vi "RSZVB Write Memory Trace Data Extended.vi"(6 "Trace Data":dbl[](array[numeric]) format="%^.3e", 7 "No of Points":i32, 8 "error in (no error)":errorcluster {"code" format="%.0x"}, 9 "Data Format (0: Unformatted)":i32(ring) items=["Unformatted", "Formatted", "Unformatted With Trace Mathematics"], 10 "Channel (Trace) (1)":i32=1, 11 "VISA session":refnum<visa-resource-name>) -> (0 "error out":errorcluster {"code" format="%.0x"}, 3 "dup VISA session":refnum<visa-resource-name>)   [LabVIEW 2011]
doc: "This VI writes a memory trace data to the instrument.\n\nRemote-control command(s):\nCALCulate<Chn>:DATA FDATa | SDATa | MDATa, <data>\nFORMat ASCII\nFORMat REAL,32\nSYSTem:COMMunicate:GPIB:SELF:RTERminator EOI"
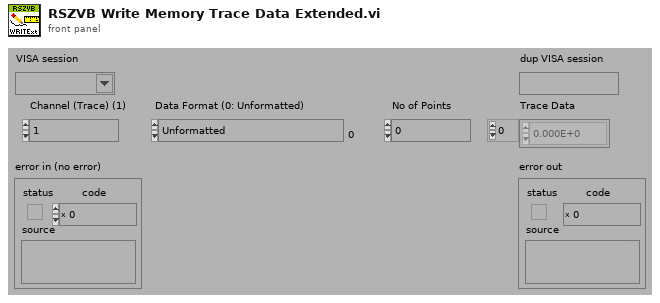
[diagram p1: front panel]
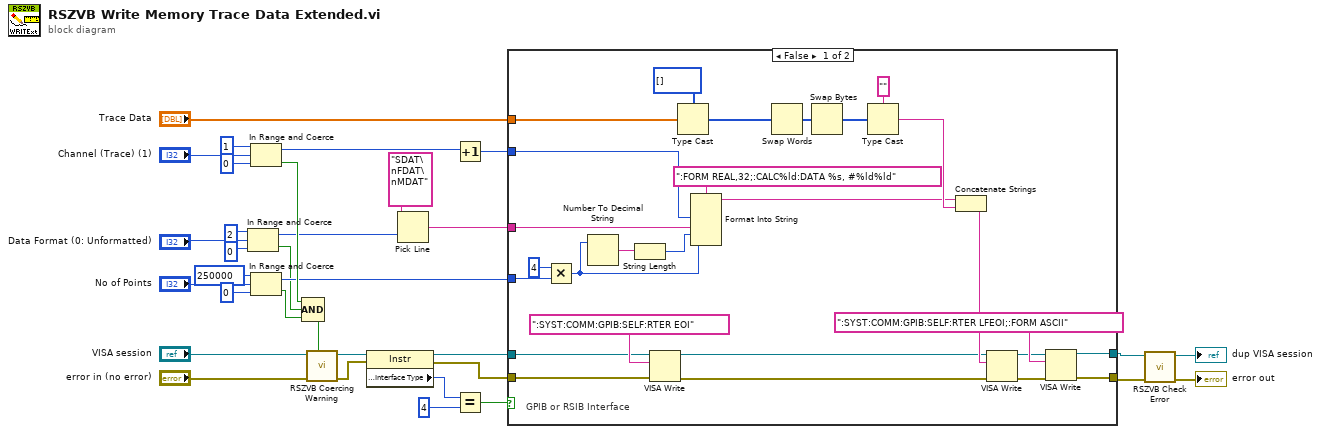
[diagram p0: block diagram]
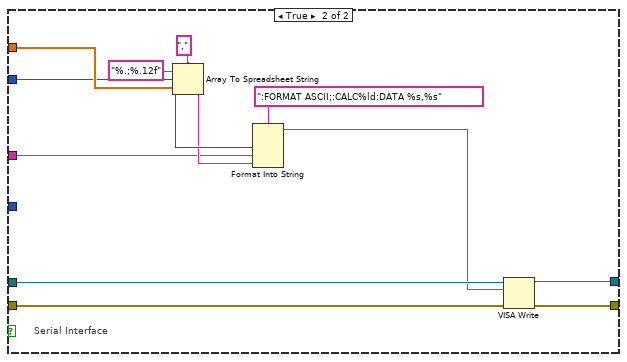
[diagram p2: hidden frame]
diagram:
  n1 = In Range and Coerce(upper limit=2, x="Data Format (0: Unformatted)", lower limit=0) -> (coerced(x)=w4:i32, In Range?=w1:bool)
  n2 = In Range and Coerce(upper limit=1, x="Channel (Trace) (1)", lower limit=0) -> (coerced(x)=w17:i32, In Range?=w21:bool)
  n3 = In Range and Coerce(upper limit=250000, x="No of Points", lower limit=0) -> (coerced(x)=w18:i32, In Range?=w8:bool)
  n4 = Compound Arithmetic op=AND(w21, w1, w8) -> (w16:bool)
  n5 = call "RSZVB Coercing Warning.vi"("In Range?"=w16, "error in (no error)"="error in (no error)", "VISA session"="VISA session") -> ("error out"=w25:errorcluster, "dup VISA session"=w24:refnum<visa-resource-name>)  [unwired: 7 in]
  n6 = property class="Instr"(reference=w24, error in=w25) -> (reference out=w31:refnum<visa-resource-name>, error out=w30:errorcluster, "Interface Information:Interface Type"=w33:u16)
  n7 = Pick Line(multi-line string="SDAT\nFDAT\nMDAT", line index=w4) -> (output string=w2:string)  [unwired: 1 in]
  n8 = Increment(x=w17) -> (x+1=w28:i32)
  n9 = Equal?(x=w33, y=u16 4) -> (x = y?=w29:bool)
  n10 = case shown="False" w29 {
    tunnel: [w58 w71] -> w26
    tunnel: [w57 w72] -> w27
    tunnel: w18 -> [w56 _]
    tunnel: "Trace Data" -> [w54 w65]
    tunnel: w30 -> [w46 w69]
    tunnel: w31 -> [w45 w70]
    tunnel: w28 -> [w37 w63]
    tunnel: w2 -> [w34 w61]
    frame False {
      # "GPIB or RSIB Interface"
      n11 = Multiply(x=u32 4, y=w56) -> (x*y=w35:u32)
      n12 = Number To Decimal String(number=w35) -> (decimal integer string=w41:string)  [unwired: 1 in]
      n13 = String Length(string=w41) -> (length=w36:i32)
      n14 = VISA Write(VISA resource name=w45, write buffer=":SYST:COMM:GPIB:SELF:RTER EOI", error in (no error)=w46) -> (VISA resource name out=w50:refnum<visa-resource-name>, error out=w47:errorcluster)  [unwired: 1 out]
      n15 = Type Cast(type=i32[] [], x=w54) -> (*(type *) &x=w59:i32[])
      n16 = Format Into String(format string=":FORM REAL,32;:CALC%ld:DATA %s, #%ld%ld", w37, w34, w36, w35) -> (resulting string=w42:string)  [unwired: 2 in, 1 out]
      n17 = Swap Words(1:w59) -> (0:w40:i32[])
      n18 = Swap Bytes(anything=w40) -> (byte swapped=w60:i32[])
      n19 = Type Cast(type="", x=w60) -> (*(type *) &x=w43:string)
      n20 = Concatenate Strings(w42, w43) -> (w55:string)
      n21 = VISA Write(VISA resource name=w50, write buffer=w55, error in (no error)=w47) -> (VISA resource name out=w49:refnum<visa-resource-name>, error out=w48:errorcluster)  [unwired: 1 out]
      n22 = VISA Write(VISA resource name=w49, write buffer=":SYST:COMM:GPIB:SELF:RTER LFEOI;:FORM ASCII", error in (no error)=w48) -> (VISA resource name out=w57:refnum<visa-resource-name>, error out=w58:errorcluster)  [unwired: 1 out]
    }
    frame True {
      # "Serial Interface"
      n23 = Array To Spreadsheet String(delimiter (Tab)=",", array=w65, 3:"%.;%.12f" ("format string")) -> (spreadsheet string=w62:string)
      n24 = Format Into String(format string=":FORMAT ASCII;:CALC%ld:DATA %s,%s", w63, w61, w62) -> (resulting string=w64:string)  [unwired: 2 in, 1 out]
      n25 = VISA Write(VISA resource name=w70, write buffer=w64, error in (no error)=w69) -> (VISA resource name out=w72:refnum<visa-resource-name>, error out=w71:errorcluster)  [unwired: 1 out]
    }
  }
  n26 = call "RSZVB Check Error.vi"("error in (no error)"=w26, "VISA session"=w27) -> ("error out"=→"error out":errorcluster, "dup VISA session"=→"dup VISA session":refnum<visa-resource-name>)  [unwired: 8 in]
